vi "Half_Adder_sub.vi"(10 "z":bool, 11 "Boolean 3":bool) -> (2 "Boolean":bool, 3 "Boolean 2":bool)   [LabVIEW 2024]
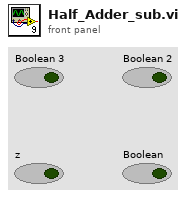
[diagram p1: front panel]
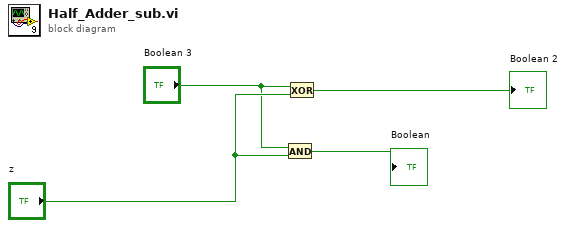
[diagram p0: block diagram]
diagram:
  n1 = And(x="Boolean 3", y="z") -> (x .and. y?=→"Boolean":bool)
  n2 = Exclusive Or(1:"z", 2:"Boolean 3") -> (0:→"Boolean 2":bool)
